vi "HardwareMessage.vi"() -> ()   [LabVIEW 2017]
uses:
  hardwareMessage.ctl
panel:
  in  "HardwareMessage":T1
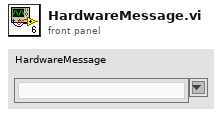
[diagram p1: front panel]
types:
  T1 = typedef "hardwareMessage.ctl" = string
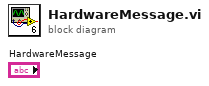
[diagram p0: block diagram]
diagram:
